vi "read_channels.vi"(5 "postDAQ  wait ms":u32=12, 7 "preDAQ  wait ms":u32=25, 8 "error in":T1, 11 "K6517 GPIB Address":string) -> (0 "error out":T1, 2 "data":dbl[](array[numeric]), 3 "K6517 GPIB Address out":string)   [LabVIEW 2024]
panel:
  out "ch3":dbl format="%.6e"
  out "ch2":dbl format="%.6e"
  out "ch1":dbl format="%.6e"
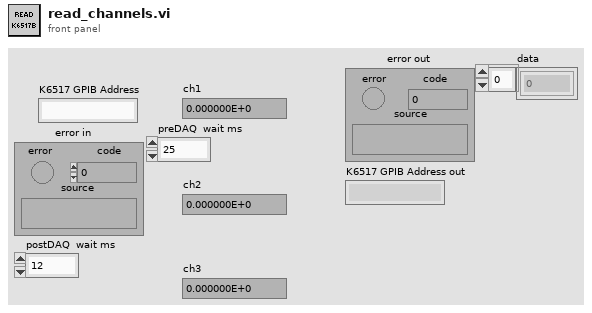
[diagram p1: front panel]
types:
  T1 = cluster{"error":bool, "code":i32, "source":string}
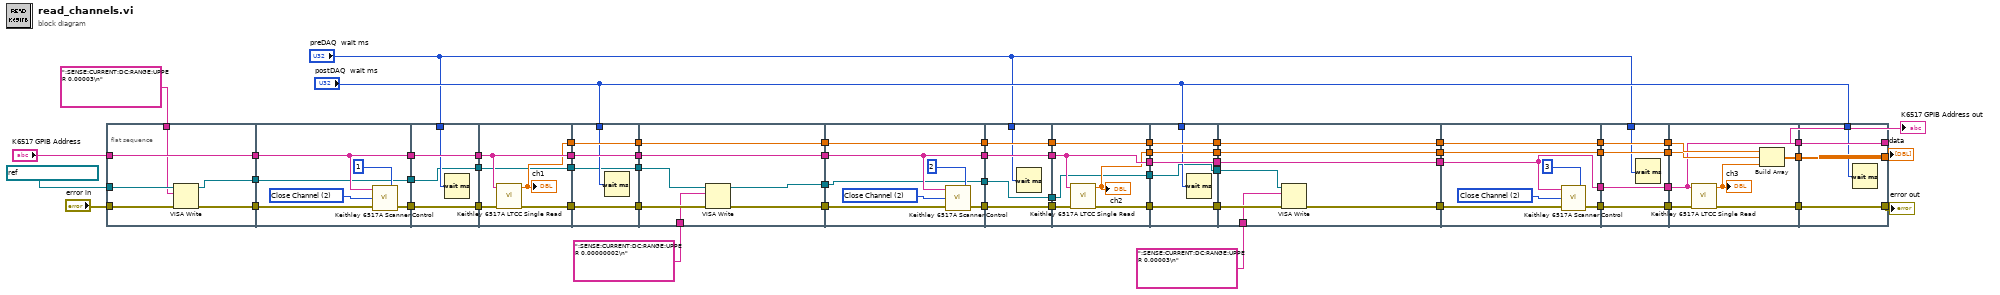
[diagram p0: block diagram]
diagram:
  n1 = flat-sequence {
    tunnel: "error in" -> [w70]
    tunnel: "K6517 GPIB Address" -> [w71]
    tunnel: [w71] -> w30
    tunnel: [w69] -> w29
    tunnel: refnum<visa-resource-name> "GPIB0::27::INSTR" ("VISA resource name") -> [w68]
    tunnel: ":SENSE:CURRENT:DC:RANGE:UPPER 0.00003\n" -> [w67]
    tunnel: [w66] -> w20
    tunnel: [w77] -> w63
    tunnel: [w73] -> w62
    tunnel: w30 -> [w77]
    tunnel: w29 -> [w76]
    tunnel: w20 -> [w72]
    tunnel: [w72] -> w19
    tunnel: w63 -> [w81]
    tunnel: [w81] -> w61
    tunnel: w62 -> [w80]
    tunnel: [w80] -> w60
    tunnel: "preDAQ  wait ms" -> [w79]
    tunnel: w19 -> [w78]
    tunnel: [w78] -> w18
    tunnel: w61 -> [w86]
    tunnel: [w86] -> w59
    tunnel: w60 -> [w85]
    tunnel: [w84] -> w58
    tunnel: [w83] -> w57
    tunnel: w18 -> [w82]
    tunnel: [w82] -> w17
    tunnel: w59 -> [w91]
    tunnel: [w91] -> w28
    tunnel: w58 -> [w90]
    tunnel: [w90] -> w26
    tunnel: w57 -> [w89]
    tunnel: [w89] -> w24
    tunnel: "postDAQ  wait ms" -> [w88]
    tunnel: w17 -> [w87]
    tunnel: [w87] -> w16
    tunnel: w28 -> [w98]
    tunnel: [w98] -> w27
    tunnel: w26 -> [w97]
    tunnel: [w95] -> w25
    tunnel: w24 -> [w96]
    tunnel: [w96] -> w23
    tunnel: w16 -> [w94]
    tunnel: ":SENSE:CURRENT:DC:RANGE:UPPER 0.00000002\n" -> [w93]
    tunnel: [w92] -> w6
    tunnel: w27 -> [w105]
    tunnel: [w105] -> w56
    tunnel: w25 -> [w104]
    tunnel: w23 -> [w103]
    tunnel: [w103] -> w55
    tunnel: [w100] -> w54
    tunnel: w6 -> [w99]
    tunnel: [w99] -> w5
    tunnel: w56 -> [w110]
    tunnel: [w110] -> w53
    tunnel: w55 -> [w109]
    tunnel: [w109] -> w52
    tunnel: w54 -> [w108]
    tunnel: [w108] -> w51
    tunnel: "preDAQ  wait ms" -> [w107]
    tunnel: w5 -> [w106]
    tunnel: [w106] -> w4
    tunnel: w53 -> [w116]
    tunnel: [w116] -> w50
    tunnel: w52 -> [w115]
    tunnel: [w115] -> w49
    tunnel: w51 -> [w114]
    tunnel: [w113] -> w48
    tunnel: [w112] -> w47
    tunnel: w4 -> [w111]
    tunnel: [w111] -> w3
    tunnel: w50 -> [w122]
    tunnel: [w122] -> w14
    tunnel: w49 -> [w121]
    tunnel: [w121] -> w12
    tunnel: w48 -> [w120]
    tunnel: [w120] -> w10
    tunnel: w47 -> [w119]
    tunnel: [w119] -> w8
    tunnel: "postDAQ  wait ms" -> [w118]
    tunnel: w3 -> [w117]
    tunnel: [w117] -> w2
    tunnel: w14 -> [w129]
    tunnel: [w129] -> w13
    tunnel: w12 -> [w128]
    tunnel: [w128] -> w11
    tunnel: w10 -> [w127]
    tunnel: [w125] -> w9
    tunnel: w8 -> [w126]
    tunnel: [w126] -> w7
    tunnel: w2 -> [w124]
    tunnel: ":SENSE:CURRENT:DC:RANGE:UPPER 0.00003\n" -> [w123]
    tunnel: w13 -> [w136]
    tunnel: [w136] -> w46
    tunnel: w11 -> [w135]
    tunnel: [w135] -> w44
    tunnel: w9 -> [w134]
    tunnel: w7 -> [w133]
    tunnel: [w133] -> w42
    tunnel: [w130] -> w40
    tunnel: w46 -> [w141]
    tunnel: [w141] -> w45
    tunnel: w44 -> [w140]
    tunnel: [w140] -> w43
    tunnel: w42 -> [w139]
    tunnel: [w139] -> w41
    tunnel: w40 -> [w138]
    tunnel: [w138] -> w39
    tunnel: "preDAQ  wait ms" -> [w137]
    tunnel: w45 -> [w142]
    tunnel: w43 -> [w147]
    tunnel: w41 -> [w146]
    tunnel: w39 -> [w145]
    tunnel: [w144] -> w35
    tunnel: [w143] -> w34
    tunnel: [w142] -> w33
    tunnel: [w150] -> w36
    tunnel: [w151] -> w37
    tunnel: [w152] -> w38
    tunnel: w35 -> [w152]
    tunnel: w34 -> [w151]
    tunnel: w33 -> [w150]
    tunnel: "postDAQ  wait ms" -> [w149]
    frame #0 {
      n2 = VISA Write(VISA resource name=w68, write buffer=w67, error in (no error)=w70) -> (VISA resource name out=w66:refnum<visa-resource-name>, error out=w69:errorcluster)  [unwired: 1 out]
    }
    frame #1 {
      w74 = u16 2 items=["Open All", "Open Channel", "Close Channel", "Scan List"] ("Scanner Control")
      n3 = call "Keithley 6517A Scanner Control.vi"("Open / Close Internal Scanner Channel"=i16 1, "error in"=w76, "Scanner Control"=w74, "GPIB address"=w77) -> ("error out"=w73:T1)  [unwired: 1 in]
    }
    frame #2 {
      n4 = Wait (ms)(milliseconds to wait=w79) -> ()  [unwired: 1 out]
    }
    frame #3 {
      n5 = call "Keithley 6517A LTCC Single Read.vi"("error in"=w85, "GPIB address"=w86) -> ("error out"=w84:T1, "measurement"=w83:dbl)  [unwired: 2 in, 6 out]
      "ch1" <- w83
    }
    frame #4 {
      n6 = Wait (ms)(milliseconds to wait=w88) -> ()  [unwired: 1 out]
    }
    frame #5 {
      n7 = VISA Write(VISA resource name=w94, write buffer=w93, error in (no error)=w97) -> (VISA resource name out=w92:refnum<visa-resource-name>, error out=w95:errorcluster)  [unwired: 1 out]
    }
    frame #6 {
      w101 = u16 2 items=["Open All", "Open Channel", "Close Channel", "Scan List"] ("Scanner Control")
      n8 = call "Keithley 6517A Scanner Control.vi"("Open / Close Internal Scanner Channel"=i16 2, "error in"=w104, "Scanner Control"=w101, "GPIB address"=w105) -> ("error out"=w100:T1)  [unwired: 1 in]
    }
    frame #7 {
      n9 = Wait (ms)(milliseconds to wait=w107) -> ()  [unwired: 1 out]
    }
    frame #8 {
      n10 = call "Keithley 6517A LTCC Single Read.vi"("error in"=w114, "GPIB address"=w116) -> ("error out"=w113:T1, "measurement"=w112:dbl)  [unwired: 2 in, 6 out]
      "ch2" <- w112
    }
    frame #9 {
      n11 = Wait (ms)(milliseconds to wait=w118) -> ()  [unwired: 1 out]
    }
    frame #10 {
      n12 = VISA Write(VISA resource name=w124, write buffer=w123, error in (no error)=w127) -> (error out=w125:errorcluster)  [unwired: 2 out]
    }
    frame #11 {
      w131 = u16 2 items=["Open All", "Open Channel", "Close Channel", "Scan List"] ("Scanner Control")
      n13 = call "Keithley 6517A Scanner Control.vi"("Open / Close Internal Scanner Channel"=i16 3, "error in"=w134, "Scanner Control"=w131, "GPIB address"=w136) -> ("error out"=w130:T1)  [unwired: 1 in]
    }
    frame #12 {
      n14 = Wait (ms)(milliseconds to wait=w137) -> ()  [unwired: 1 out]
    }
    frame #13 {
      n15 = call "Keithley 6517A LTCC Single Read.vi"("error in"=w145, "GPIB address"=w142) -> ("error out"=w144:T1, "measurement"=w148:dbl)  [unwired: 2 in, 6 out]
      "ch3" <- w148
      n16 = Build Array(w147, w146, w148) -> (w143:dbl[])
    }
    frame #14 {
      n17 = Wait (ms)(milliseconds to wait=w149) -> ()  [unwired: 1 out]
    }
  }
  "error out" <- w38
  "data" <- w37
  "K6517 GPIB Address out" <- w36
